vi "singlestep.vi"(8 "error in (no error)":errorcluster, 11 "MSCU":refnum<class "MSCU.lvclass">) -> (0 "error out":errorcluster, 2 "?":string, 3 "MSCU":refnum<class "MSCU.lvclass">)   [LabVIEW 2019, in "MSCU.lvclass"]
uses:
  MSCU.lvclass
  MSCU.lvclass/MSCU.ctl
panel:
  in  "Direction":string(combo)
  in  "Axis":string(combo)
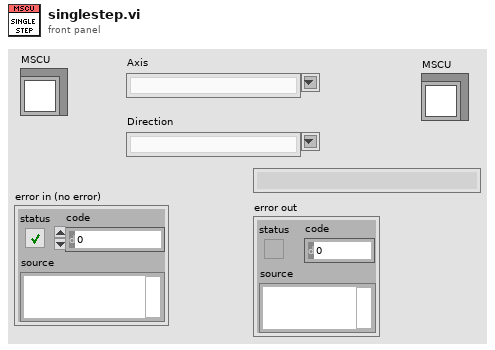
[diagram p1: front panel]
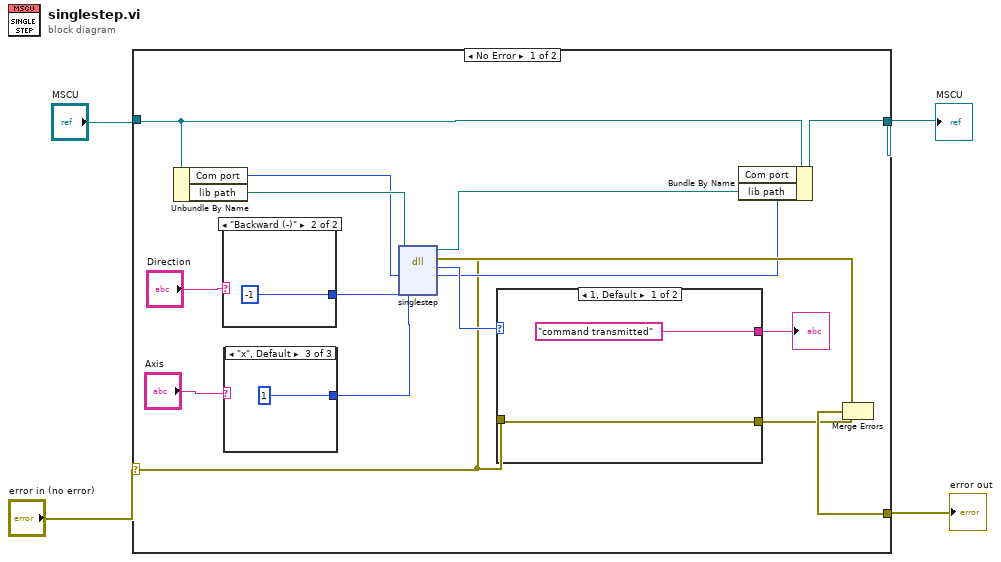
[diagram p0: block diagram]
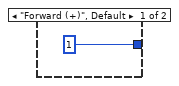
[diagram p2: hidden frame]
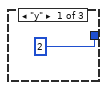
[diagram p3: hidden frame]
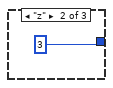
[diagram p4: hidden frame]
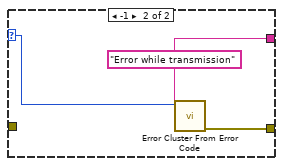
[diagram p5: hidden frame]
diagram:
  n1 = case shown="No Error" "error in (no error)" {
    selector: "error in (no error)" -> [w9 w31]
    tunnel: "MSCU" -> [w13 w32]
    tunnel: [w12 w31] -> w3
    tunnel: [w11 w32] -> w2
    frame No Error {
      n2 = Unbundle By Name(w13) -> ("Com port"=w17:i32, "lib path"=w18:path)
      n3 = case shown="\"Backward (-)\"" "Direction" {
        tunnel: [1 -1 ("Channel")] -> w5
        frame "Forward (+)", Default {
        }
        frame "Backward (-)" {
        }
      }
      n4 = case shown="\"x\", Default" "Axis" {
        tunnel: [2 3 1 ("Direction")] -> w7
        frame "y" {
        }
        frame "z" {
        }
        frame "x", Default {
        }
      }
      n5 = dll-call lib="C:/Program Files (x86)/Nanonis/SPM Controller/data/MSCU.dll" fn="singlestep"(path in=w18, error in=w9, "Comport"=w17, "Channel"=w7, "Direction"=w5) -> (path out=w19:path, error out=w20:errorcluster, "return type"=w16:i32, "Comport"=w14:i32)  [unwired: 3 in]
      n6 = case shown="1, Default" w16 {
        selector: w16 -> [_ w30]
        tunnel: ["command transmitted" w29] -> w15
        tunnel: [w26 w28] -> w10
        tunnel: w9 -> [w26 _]
        frame 1, Default {
        }
        frame -1 {
          w29 = "Error while transmission"
          n7 = call <vilib>:"Error Cluster From Error Code.vi"("error message (\"\")"=w29, "error code (0)"=w30) -> ("error out"=w28:errorcluster)  [unwired: 7 in]
        }
      }
      "?" <- w15
      n8 = Bundle By Name(cluster=w13, "Com port"=w14, "lib path"=w19) -> (w11:refnum<class "MSCU.lvclass">)
      n9 = Merge Errors(w20, w10) -> (w12:errorcluster)
    }
    frame Error {
    }
  }
  "MSCU" <- w2
  "error out" <- w3
